vi "matrici_v0_v42.vi"() -> ()   [LabVIEW 2009]
uses:
  <vilib>/Math Plots/3D Math Plots/3D Surface/3D Surface XCtrl/3D Surface.xctl
  <vilib>/Math Plots/3D Math Plots/3D Surface/3D Surface Datatype/3D Surface Datatype.lvclass
  <vilib>/Math Plots/3D Math Plots/3D Surface/3D Surface Datatype/Public/Plot Helper (Vector).vi
  <vilib>/Analysis/Matrix/Numeric/Conversions/Array To Matrix - RA2.vi
  <vilib>/Analysis/Matrix/NI_Matrix.lvlib
panel:
  out "3D Surface":refnum<class "3D Plot Datatype.lvclass">[](xcontrol)
  out "X":dbl=1.7725375626043396
  out "y":dbl=1.7725375626043396
  in  "stop":bool
  in  "Domeniul de definitie x,y":dbl(slide)=3.545075125208681 scale=0.5..10.0
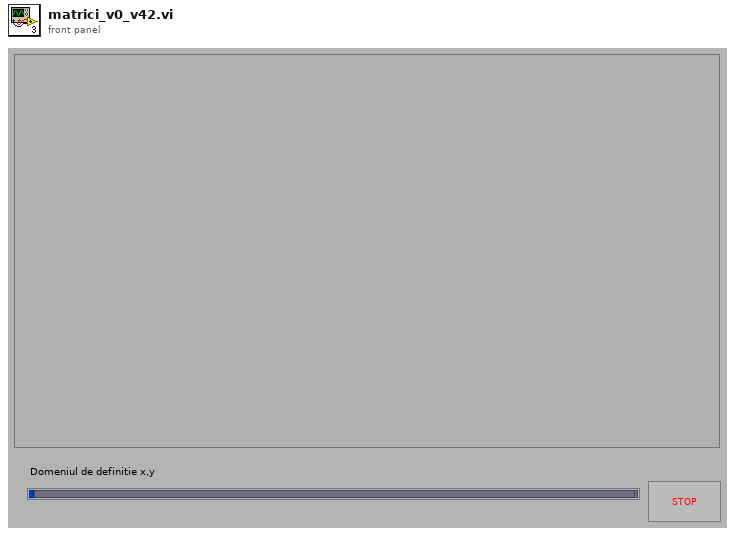
[diagram p1: front panel]
types:
  T1 = typedef "NI_Matrix.lvlib/RealMatrix.ctl" = dbl[][]
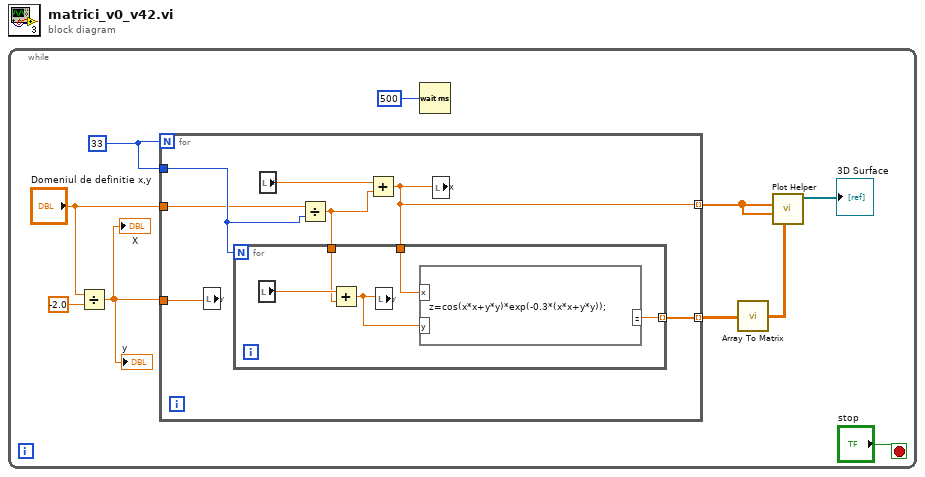
[diagram p0: block diagram]
diagram:
  n1 = while {
    stop <- "stop" stop-if-true
    w4 = 33
    n2 = Divide(x="Domeniul de definitie x,y", y=-2.0) -> (x/y=w1:dbl)
    "X" <- w1
    "y" <- w1
    n3 = for {
      N: w4 -> [_]
      tunnel: [w16] -> w8 mode=indexing
      tunnel: [w15] -> w9 mode=indexing
      tunnel: w4 -> [w14]
      tunnel: w1 -> [w12]
      tunnel: "Domeniul de definitie x,y" -> [w11]
      n4 = local write "y"(w12) -> ()
      n5 = local read "X"() -> (w17:dbl)
      n6 = Divide(x=w11, y=w14) -> (x/y=w13:dbl)
      n7 = Add(x=w17, y=w13) -> (x+y=w16:dbl)
      n8 = for {
        N: w14 -> [_]
        tunnel: w16 -> [w21]
        tunnel: [w19] -> w15 mode=indexing
        tunnel: w13 -> [w18]
        n9 = local read "y"() -> (w22:dbl)
        n10 = Add(x=w22, y=w18) -> (x+y=w20:dbl)
        n11 = local write "y"(w20) -> ()
        n12 = formula code="z=cos(x*x+y*y)*exp(-0.3*(x*x+y*y));"("x"=w21, "y"=w20) -> ("z"=w19:dbl)
      }
      n13 = local write "X"(w16) -> ()
    }
    n14 = Wait (ms)(milliseconds to wait=500) -> ()  [unwired: 1 out]
    n15 = call-poly <vilib>:"Array To Matrix.vi"("Real 2D Array"=w9) -> ("Real Matrix"=w10:T1)
    n16 = call-poly <vilib>:"Plot Helper.vi"("z matrix"=w10, "y vector"=w8, "x vector"=w8) -> ("3D Plot lvclass Array out"=→"3D Surface":refnum<class "3D Plot Datatype.lvclass">[])  [unwired: 3 in, 5 out]
  }
